vi "TeleWrite.vi"() -> ()   [LabVIEW 2017]
uses:
  <vilib>/Platform/TimedLoop/XDataNode/timing_clust.ctl
  <vilib>/Platform/TimedLoop/XDataNode/nitl_modes.ctl
  <vilib>/Platform/TimedLoop/XDataNode/wakeup.ctl
  <vilib>/platform/TimedLoop/XDataNode/XDataNode.xnode
  <vilib>/Platform/TimedLoop/XDataNode/XDNodeRunTimeDep.lvlib
panel:
  out "error out":errorcluster
  in  "Port":u16=9000
  in  "IP":string="10.25.37.100"
  in  "Stop":bool
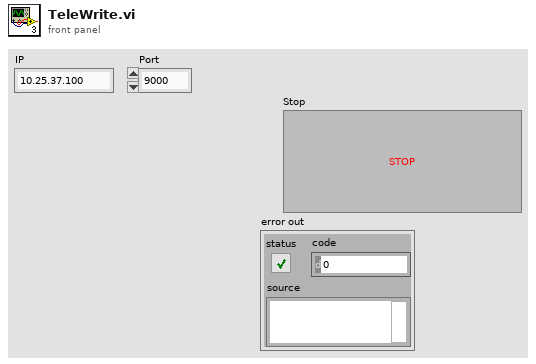
[diagram p1: front panel]
types:
  T1 = typedef "XDNodeRunTimeDep.lvlib/timing_clust.ctl" = cluster{"Expected End [f-1]":u64, "Actual End [f-1]":u64, "Finished Late? [f-1]":bool, "Expected End [i-1]":u64, "Actual End [i-1]":u64, "Finished Late? [i-1]":bool, "Expected Start [i]":u64, "Actual Start [i]":u64, "Expected Start [f]":u64, "Actual Start [f]":u64, "Source Name":string, "Structure Name":string, "Period":i64, "Deadline":i64, "Offset":i64, "Start":i64, "Priority":i32, "Timeout":i32, "Mode":T2, "Wakeup Reason":T3, "Error":errorcluster, "Source Type":string, "Secondary Source Type":string, "Global End Time":u64, "Global Start Time":u64, "Frame Duration":u64, "Iteration Duration":u64, "Assigned CPU":i32, "I/O Scan Engine Mode":u32}
  T2 = typedef "XDNodeRunTimeDep.lvlib/nitl_modes.ctl" = enum32{"No Change", "Process missed periods, maintain original phase", "Discard missed periods, maintain original phase", "Process missed periods, ignore original phase", "Discard missed periods, ignore original phase"}
  T3 = typedef "XDNodeRunTimeDep.lvlib/wakeup.ctl" = enum32{"Normal", "Aborted", "Asynchronous wakeup", "Timing source error", "Timed loop error", "Timeout"}
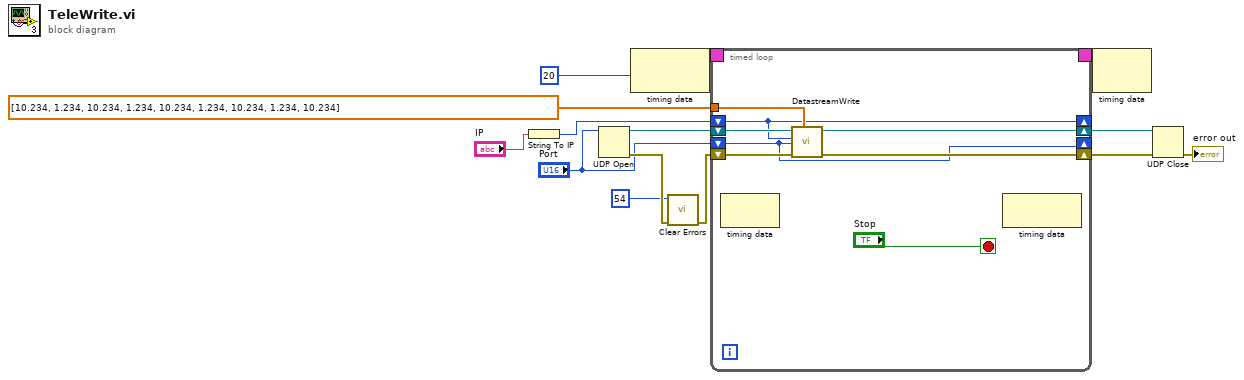
[diagram p0: block diagram]
diagram:
  n1 = String To IP(1:"IP") -> (0:w2:u32)
  n2 = UDP Open(11:"Port") -> (port=w7:refnum<k16>, 0:w4:errorcluster)  [unwired: 4 in, 1 out]
  n3 = node-c288(i64 20 ("Period")) -> (w12:T1)
  n4 = call <vilib>:"Clear Errors.vi"("error in (no error)"=w4, "specific error code to clear (0: all)"=54) -> ("error out"=w5:errorcluster)  [unwired: 4 in, 1 out]
  n5 = timed-loop {
    tunnel: dbl[] [10.234, 1.234, 10.234, 1.234, 10.234, 1.234, 10.234, 1.234, 10.234] ("Data") -> [w21]
    timing: w12 -> [_]
    timing-out: [_] -> w11
    shift-right: [w19] -> w8
    shift-left: w7 -> [w18]
    shift-right: [w20] -> w9
    shift-left: w5 -> [w17]
    shift-right: [w16] -> _
    shift-left: "Port" -> [w16]
    shift-right: [w15] -> _
    shift-left: w2 -> [w15]
    stop <- "Stop" stop-if-true
    n6 = node-c288() -> ()  [unwired: 1 in, 1 out]
    n7 = call "DatastreamWrite.vi"("Data"=w21, "error in (no error)"=w17, "port or service name"=w16, "address"=w15, "connection ID"=w18) -> ("error out"=w20:errorcluster, "connection ID out"=w19:refnum<k16>)  [unwired: 5 in]
    n8 = node-c288() -> ()  [unwired: 1 in, 1 out]
  }
  n9 = node-c288(w11) -> ()  [unwired: 1 out]
  n10 = UDP Close(connection ID=w8, 8:w9) -> (error out=→"error out":errorcluster)  [unwired: 1 out]
